vi "Create User Error Codes File.vi"(6 "MetaDataObj":refnum<class "MetaDataObj.lvclass">, 8 "error in (no error)":errorcluster, 11 "Project":refnum<vi>) -> (0 "error out":errorcluster, 3 "dup Project":refnum<vi>)   [LabVIEW 2016, in "NI_NPW_Project Copying.lvlib"]
uses:
  <resource>/dialog/NewProjectWizard/Project Copying/NI_NPW_Project Copying.lvlib
  <resource>/dialog/NewProjectWizard/MetaDataObj/MetaDataObj.lvclass
  <vilib>/Utility/traverseref.llb/TRef TravTarget.ctl
  <vilib>/Utility/traverseref.llb/VI Scripting - Traverse.lvlib
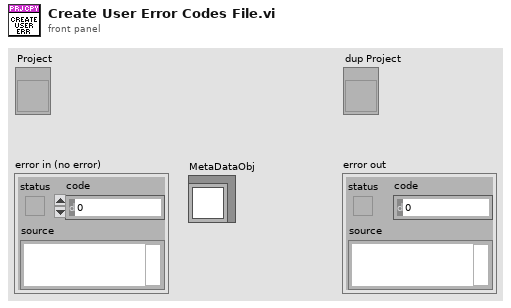
[diagram p1: front panel]
types:
  T1 = typedef "TRef TravTarget.ctl" = enum16{"FP", "BD", "Other"}
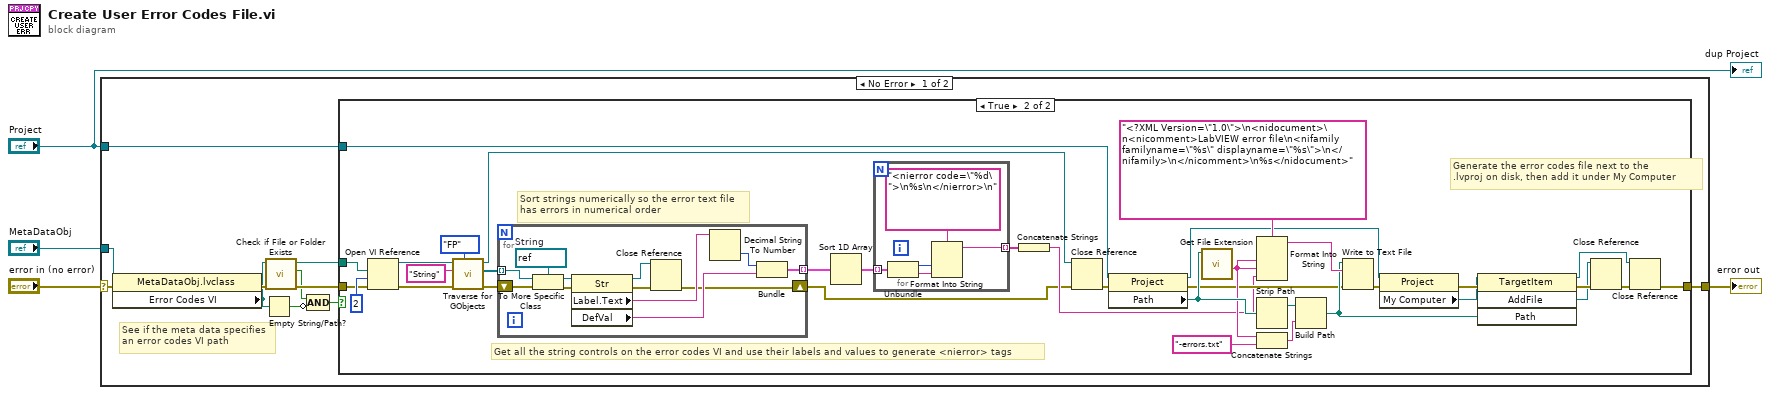
[diagram p0: block diagram]
diagram:
  n1 = case shown="No Error" "error in (no error)" {
    selector: "error in (no error)" -> [w13 w69]
    tunnel: "Project" -> [w15 _]
    tunnel: [w6 w69] -> w2
    tunnel: "MetaDataObj" -> [w14 _]
    frame No Error {
      # "See if the meta data specifies\nan error codes VI path"
      n2 = property class="MetaDataObj.lvclass"(reference=w14, error in=w13) -> (error out=w12:errorcluster, "Error Codes VI"=w9:path)  [unwired: 1 out]
      n3 = Empty String/Path?(string/path=w9) -> (empty?=w8:bool)
      n4 = call <vilib>:"Check if File or Folder Exists.vi"("error in (no error)"=w12, "path"=w9) -> ("error out"=w11:errorcluster, "file or folder exists?"=w10:bool, "dup path"=w5:path)  [unwired: 7 in]
      n5 = Compound Arithmetic op=AND(w10, invert w8) -> (w7:bool)
      n6 = case shown="True" w7 {
        tunnel: w15 -> [_ w49]
        tunnel: w11 -> [w16 w27]
        tunnel: [w16 w17] -> w6
        tunnel: w5 -> [_ w43]
        frame False {
          # "No error codes VI"
        }
        frame True {
          # "Sort strings numerically so the error text file\nhas errors in numerical order"
          # "Generate the error codes file next to the\n.lvproj on disk, then add it under My Computer"
          # "Get all the string controls on the error codes VI and use their labels and values to generate <nierror> tags"
          n7 = Open VI Reference(vi path=w43, options=2, error in (no error)=w27) -> (vi reference=w40:refnum<vi>, error out=w41:errorcluster)  [unwired: 3 in]
          n8 = call <vilib>:"Traverse for GObjects.vi"("Traverse Target"=TRef_TravTarget."FP", "error in (no error)"=w41, "Class Name"="String", "VI Refnum"=w40) -> ("error out"=w24:errorcluster, "References"=w23:refnum<vi>[], "dup VI Refnum"=w37:refnum<vi>)  [unwired: 4 in, 1 out]
          n9 = for {
            shift-right: [w53] -> w18
            shift-left: w24 -> [w62]
            tunnel: w23 -> [w61] mode=indexing
            tunnel: [w55] -> w22 mode=indexing
            w63 = refnum<vi> refnum  # String
            n10 = To More Specific Class(target class=w63, reference=w61, error in=w62) -> (specific class reference=w59:refnum<vi>, error out=w60:errorcluster)
            n11 = property class="Str"(reference=w59, error in=w60) -> (reference out=w52:refnum<vi>, error out=w58:errorcluster, "Label.Text"=w57:string, "DefVal"=w54:string)
            n12 = Close Reference(reference=w52, error in (no error)=w58) -> (error out=w53:errorcluster)
            n13 = Decimal String To Number(string=w57) -> (number=w56:i32)  [unwired: 2 in, 1 out]
            n14 = Bundle(w56, "DefVal"=w54) -> (w55:cluster{i32, "DefVal":string})  [unwired: 1 in]
          }
          n15 = Sort 1D Array(array=w22) -> (sorted array=w21:cluster{i32, "DefVal":string}[])
          n16 = for {
            tunnel: w21 -> [w67] mode=indexing
            tunnel: [w64] -> w20 mode=indexing
            n17 = Unbundle(w67) -> (w66:i32, "DefVal"=w65:string)
            n18 = Format Into String(format string="<nierror code=\"%d\">\n%s\n</nierror>\n", w66, w65) -> (resulting string=w64:string)  [unwired: 2 in, 1 out]
          }
          n19 = Concatenate Strings(w20) -> (w19:string)
          n20 = Close Reference(reference=w37, error in (no error)=w18) -> (error out=w26:errorcluster)
          n21 = property class="Project"(reference=w49, error in=w26) -> (reference out=w35:refnum<vi>, error out=w25:errorcluster, "Path"=w48:path)
          n22 = call <vilib>:"Get File Extension.vi"("file"=w48) -> ("filename without extension"=w47:string)  [unwired: 6 in, 4 out]
          n23 = Format Into String(format string="<?XML Version=\"1.0\">\n<nidocument>\n<nicomment>LabVIEW error file\n<nifamily familyname=\"%s\" displayname=\"%s\">\n</nifamily>\n</nicomment>\n%s</nidocument>", w47, w47, w19) -> (resulting string=w50:string)  [unwired: 2 in, 1 out]
          n24 = Strip Path(path=w48) -> (stripped path=w45:path)  [unwired: 1 out]
          n25 = Concatenate Strings(w47, "-errors.txt" ("string")) -> (w44:string)
          n26 = Build Path(base path=w45, name or relative path=w44) -> (appended path=w31:path)
          n27 = Write to Text File(file (use dialog)=w31, text=w50, error in=w25) -> (error out=w34:errorcluster)  [unwired: 1 in, 2 out]
          n28 = property class="Project"(reference=w35, error in=w34) -> (error out=w36:errorcluster, "My Computer"=w32:refnum<vi>)  [unwired: 1 out]
          n29 = invoke class="TargetItem" method="AddFile"(reference=w32, error in=w36, "Path"=w31) -> (reference out=w28:refnum<vi>, error out=w33:errorcluster, "AddFile"=w29:refnum<vi>)  [unwired: 1 in, 1 out]
          n30 = Close Reference(reference=w29, error in (no error)=w33) -> (error out=w30:errorcluster)
          n31 = Close Reference(reference=w28, error in (no error)=w30) -> (error out=w17:errorcluster)
        }
      }
    }
    frame Error {
    }
  }
  "error out" <- w2
  "dup Project" <- "Project"
